vi "additional-csv-header.vi"(6 "CSV Data Headings":string="time (s),T1,T2,T3,T4,T5,T6,T7,T8,T9,T10,T11,T12,P1,P2,P3,P4", 7 "Additional Text Heading":string="Flow1,Flow2,Flow3,Flow4", 8 "Flow 4":dbl, 9 "Flow 3":dbl, 10 "Flow 2":dbl, 11 "Flow 1":dbl) -> (2 "new-csv-header":string)   [LabVIEW 2020]
panel:
  # "Adds additional headings and data into the CSV file"
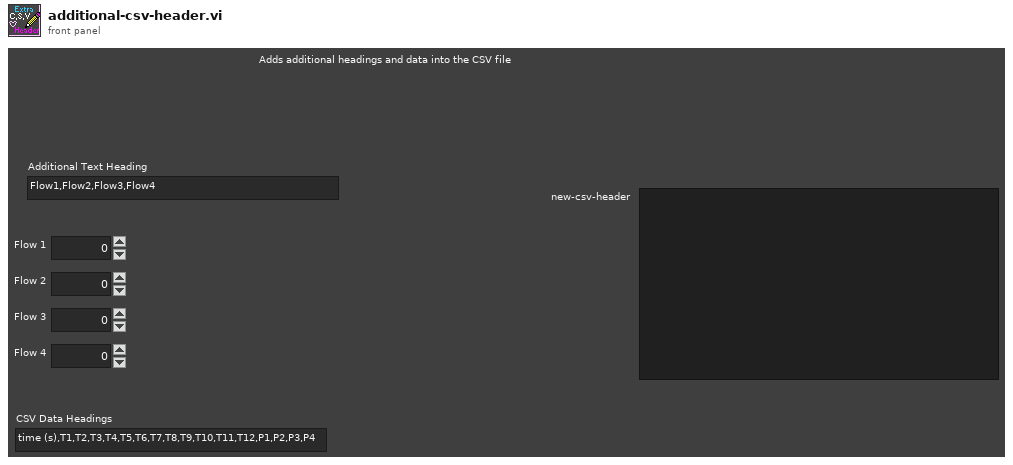
[diagram p1: front panel]
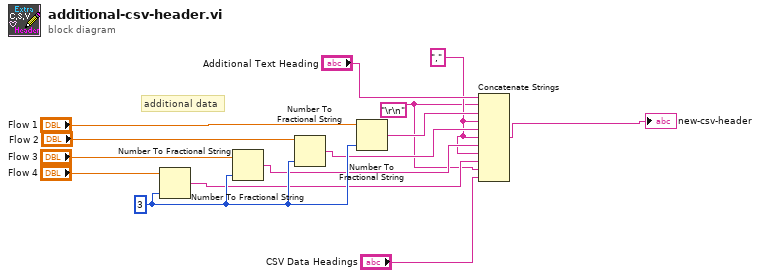
[diagram p0: block diagram]
diagram:
  w4 = "," ("string")
  w7 = i16 3 ("precision (6)")
  w2 = "\r\n"
  # "additional data"
  n1 = Number To Fractional String(number="Flow 4", precision (6)=w7) -> (F-format string=w3:string)  [unwired: 2 in]
  n2 = Number To Fractional String(number="Flow 3", precision (6)=w7) -> (F-format string=w5:string)  [unwired: 2 in]
  n3 = Number To Fractional String(number="Flow 2", precision (6)=w7) -> (F-format string=w6:string)  [unwired: 2 in]
  n4 = Number To Fractional String(number="Flow 1", precision (6)=w7) -> (F-format string=w11:string)  [unwired: 2 in]
  n5 = Concatenate Strings("Additional Text Heading", w2, w11, w4, w6, w4, w5, w4, w3, w2, "CSV Data Headings") -> (→"new-csv-header":string)
